vi "_Close Pipe.vi"(8 "error in":errorcluster, 11 "fd":u64) -> (0 "error out":errorcluster, 3 "fd out":u64)   [LabVIEW 2020, in "NI_Subprocess.lvlib" / "Subprocess.lvclass"]
uses:
  <vilib>/Subprocess/Subprocess/Subprocess.lvclass
  lviosrg.dll
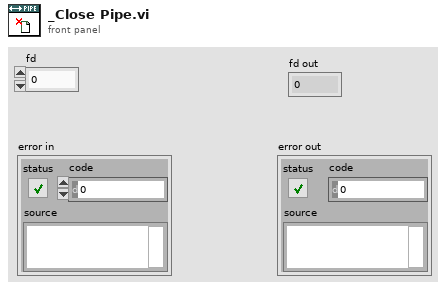
[diagram p1: front panel]
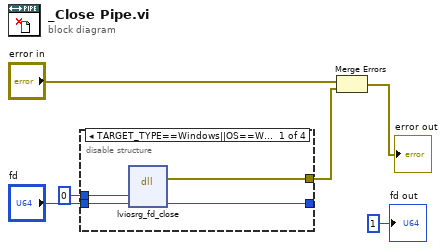
[diagram p0: block diagram]
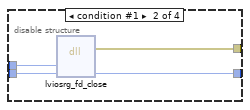
[diagram p2: hidden frame]
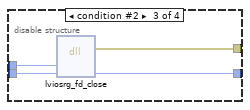
[diagram p3: hidden frame]
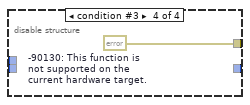
[diagram p4: hidden frame]
diagram:
  n1 = disable-structure "Conditional Disable Structure" shown="TARGET_TYPE==Windows||OS==Win" {
    disable-tunnel: "fd" -> [w10 w14 w18 _]
    disable-tunnel: [w9 w13 w17 _] -> _
    disable-tunnel: [w8 w12 w16 w19] -> w2
    disable-tunnel: 0 ("errno") -> [w7 w11 w15 _]
    frame condition #0 (active) {
      n2 = dll-call lib="lviosrg.*" fn="lviosrg_fd_close"("errno"=w7, "fd"=w10) -> (error out=w8:errorcluster, "fd"=w9:u64)  [unwired: 5 in, 1 out]
    }
    frame condition #1 {
      n3 = dll-call lib="lviosrg.*" fn="lviosrg_fd_close"("errno"=w11, "fd"=w14) -> (error out=w12:errorcluster, "fd"=w13:u64)  [unwired: 5 in, 1 out]
    }
    frame condition #2 {
      n4 = dll-call lib="lviosrg.*" fn="lviosrg_fd_close"("errno"=w15, "fd"=w18) -> (error out=w16:errorcluster, "fd"=w17:u64)  [unwired: 5 in, 1 out]
    }
    frame condition #3 {
      w19 = errorcluster {"status"=TRUE, "code"=-90130, "source"=""}  # -90130: This function is not supported on the current hardware target.
    }
  }
  n5 = Merge Errors("error in", w2) -> (→"error out":errorcluster)
  "fd out" <- u64 1 ("fd out")
